vi "Or de strings.vi"(2 "Error In":errorcluster, 3 "Datos de entrada":T1={"Current T"=0.0, "Max T"=30.0, "Min T"=10.0, "Warning"="", "Hay peligro?"=FALSE}) -> (0 "Error Out":errorcluster, 1 "Datos de salida":T1={"Current T"=0.0, "Max T"=30.0, "Min T"=10.0, "Warning"="", "Hay peligro?"=FALSE})   [LabVIEW 2016]
doc: "Revisa la temperatura actual para verificar si se sale de los limites (inferior o menor) establecidos"
uses:
  type.ctl
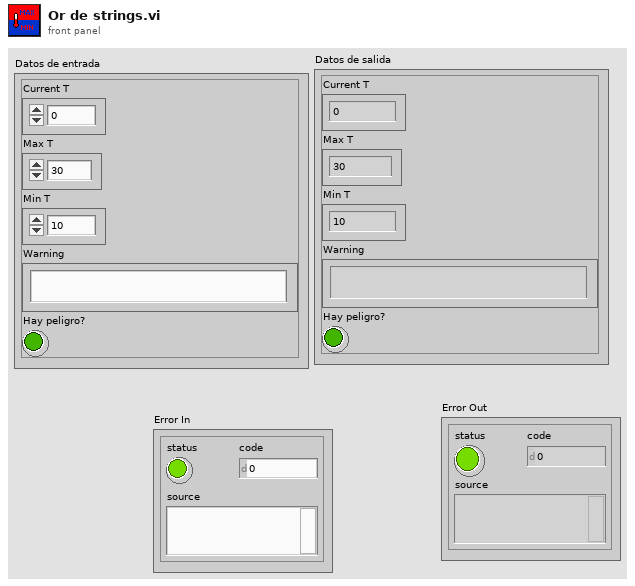
[diagram p1: front panel]
types:
  T1 = typedef "type.ctl" = cluster{"Current T":dbl, "Max T":dbl, "Min T":dbl, "Warning":string, "Hay peligro?":bool}
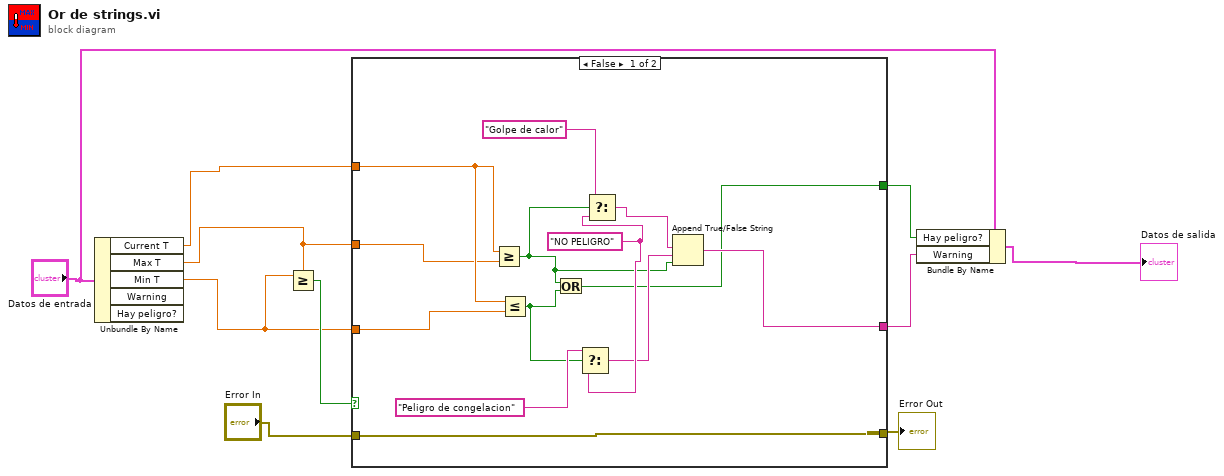
[diagram p0: block diagram]
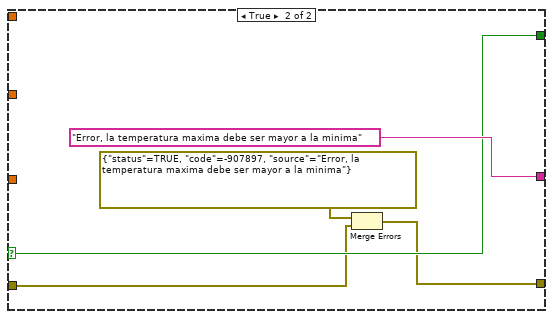
[diagram p2: hidden frame]
diagram:
  n1 = Unbundle By Name("Datos de entrada") -> ("Current T"=w2:dbl, "Max T"=w4:dbl, "Min T"=w3:dbl)  [unwired: 2 out]
  n2 = Greater Or Equal?(x=w3, y=w4) -> (x >= y?=w10:bool)
  n3 = case shown="False" w10 {
    selector: w10 -> [_ w27]
    tunnel: w3 -> [w23 _]
    tunnel: w2 -> [w22 _]
    tunnel: w4 -> [w21 _]
    tunnel: [w13 "Error, la temperatura maxima debe ser mayor a la minima" ("Warning 2")] -> w6
    tunnel: [w12 w27] -> w5
    tunnel: "Error In" -> [w11 w25]
    tunnel: [w11 w24] -> w8
    frame False {
      w18 = "NO PELIGRO"
      n4 = Greater Or Equal?(x=w22, y=w21) -> (x >= y?=w14:bool)
      n5 = Less Or Equal?(x=w22, y=w23) -> (x <= y?=w15:bool)
      n6 = Or(x=w14, y=w15) -> (x .or. y?=w12:bool)
      n7 = Select(t="Peligro de congelacion", s=w15, f=w18) -> (s? t:f=w17:string)
      n8 = Select(t="Golpe de calor", s=w14, f=w18) -> (s? t:f=w16:string)
      n9 = Append True/False String(1:w14, 2:w17, 3:w16) -> (0:w13:string)  [unwired: 1 in]
    }
    frame True {
      n10 = Merge Errors(errorcluster {"status"=TRUE, "code"=-907897, "source"="Error, la temperatura maxima debe ser mayor a la minima"} ("error constant"), w25) -> (w24:errorcluster)
    }
  }
  "Error Out" <- w8
  n11 = Bundle By Name(cluster="Datos de entrada", "Hay peligro?"=w5, "Warning"=w6) -> (→"Datos de salida":T1)
